vi "Scalar JSON text to Variant.vi"(6 "Type":T1, 8 "error in (no error)":errorcluster, 9 "Variant (Data Type)":variant, 10 "Offset (no whitespace)":i32, 11 "JSON":string) -> (0 "error out":errorcluster, 1 "Variant out":variant)   [LabVIEW 2024, in "JSONtext.lvlib"]
uses:
  JSONtext.lvlib
  Data Type.ctl
  Parsing State.ctl
  Refnum Type.ctl
  Advance past String.vi
  String Subset.vi
  Strip Quotes and Unescape.vi
  Get Number Text.vi
  NaN or null to Integer ERROR.vi
  Advance past Number.vi
  Unescape JSON string.vi
  Advance past Line Ending.vi
  Text to Timestamp.vi
  NI_Data Type.lvlib
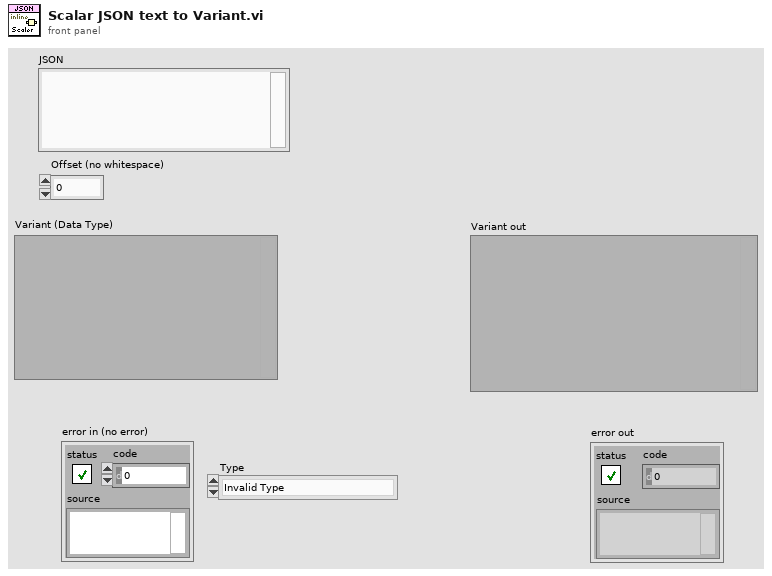
[diagram p1: front panel]
types:
  T1 = typedef "NI_Data Type.lvlib/Data Type.ctl" = enum8{"Invalid Type", "Void", "I8", "I16", "I32", "I64", "U8", "U16", "U32", "U64", "Single Float", "Double Float", "Extended Float", "Single Complex", "Double Complex", "Extended Complex", "Enum U8", "Enum U16", "Enum U32", "Enum U64", "Single Float With Unit", "Double Float With Unit", "Extended Float With Unit", "Single Complex with Unit", "Double Complex with Unit", "Extended Complex with Unit", "Boolean", "String", "Path", "Picture", "Tag", "Array", "Cluster", "Variant", "LV Variant", "Waveform", "Timestamp", "Digital Waveform", "Digital Data", "ExpressData", "Refnum", "External Data", "VI", "Poly VI", "LabVIEW Class Instance", "Fixed Point", "Set Collection", "Map Collection"}
  T2 = typedef "JSONtext.lvlib/Parsing State.ctl" = enum16{"Parser Error", "Object", "Array", "String", "Number/Other", "Leading Whitespace", "Object end", "Array end", "Value end"}
  T3 = typedef "NI_Data Type.lvlib/Refnum Type.ctl" = enum16{"NotARefnum", "UnknownRefnum", "Generic", "Datalog", "ByteStream", "Device", "Occurence", "TCPNetConnection", "Auto", "Menu", "Imaq", "Hardware", "DataSocket", "Visa", "IVI", "UDPNetConnection", "Notifier", "Queue", "Irda", "EventReg", "DotNet", "UserEvent", "Callback", "UNUSED_EMPTY_POSITION", "BlueToothNetConnection", "LVObjApp", "LVObjVI", "LVObjUnknown", "GenericClass", "UserDefinedRefnumTag", "DataValue", "RT FIFO", "TDMS File", "PythonSessionRefnum"}
  T4 = typedef "JSONtext.lvlib/JSON Value Type.ctl" = enum16{"Not a JSON Value", "JSON Object", "JSON Array", "String", "Number", "true", "false", "null"}
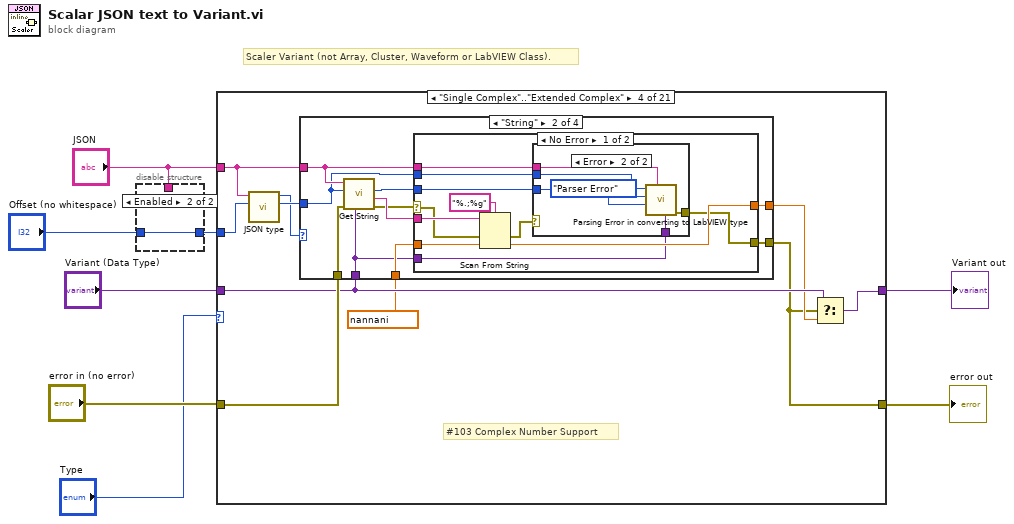
[diagram p0: block diagram]
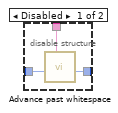
[diagram p2: hidden frame]
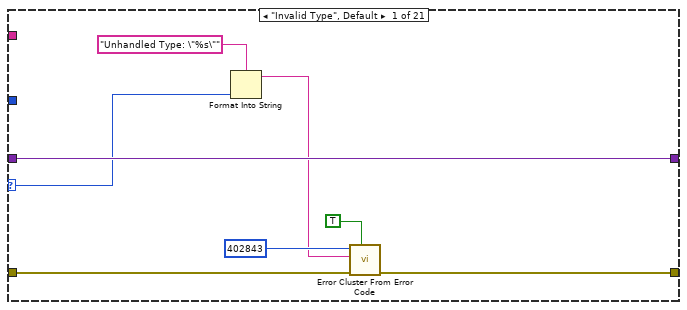
[diagram p3: hidden frame]
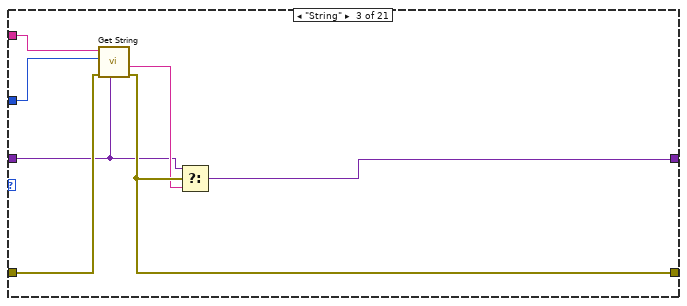
[diagram p5: hidden frame]
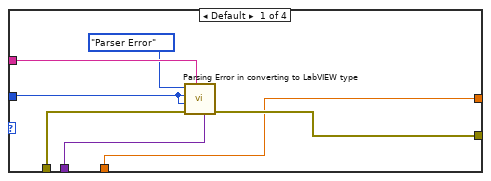
[diagram p6: hidden frame]
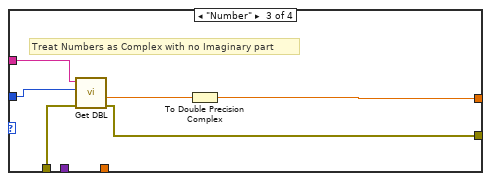
[diagram p9: hidden frame]
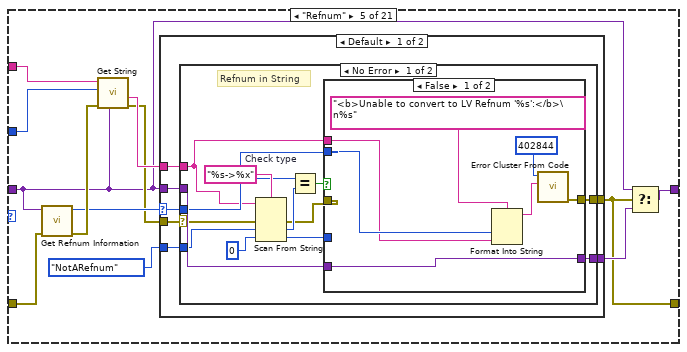
[diagram p11: hidden frame]
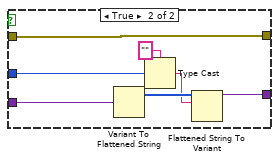
[diagram p12: hidden frame]
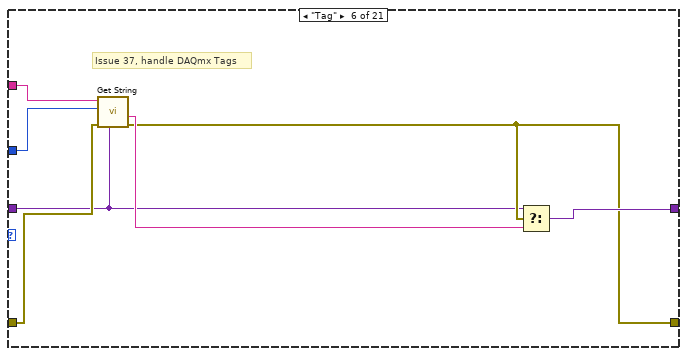
[diagram p15: hidden frame]
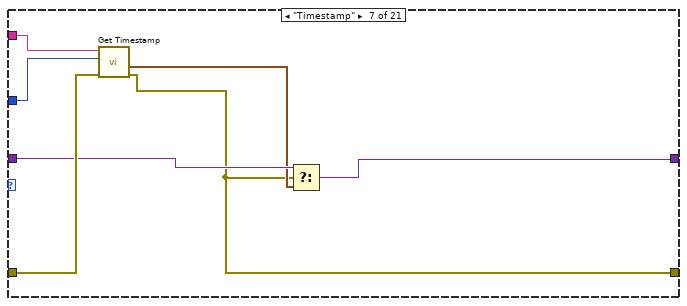
[diagram p16: hidden frame]
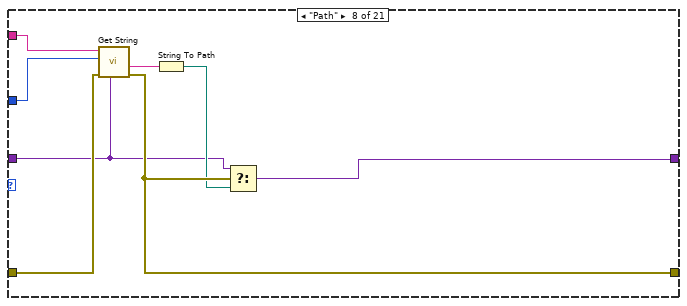
[diagram p17: hidden frame]
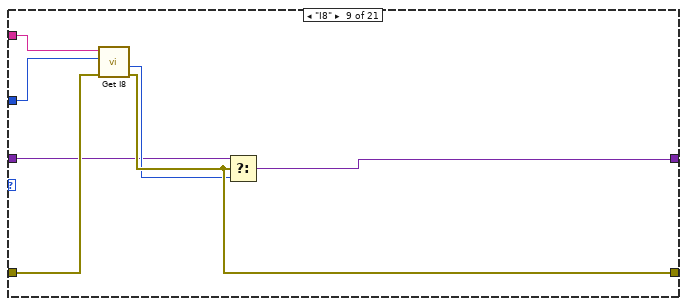
[diagram p18: hidden frame]
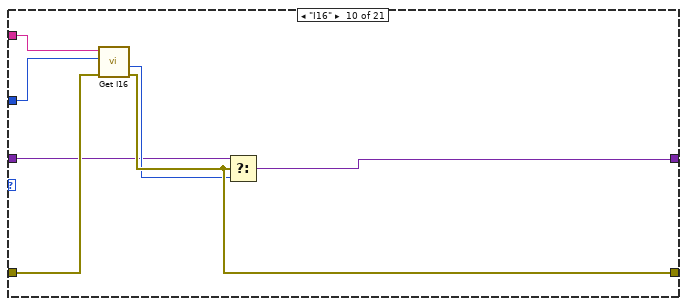
[diagram p19: hidden frame]
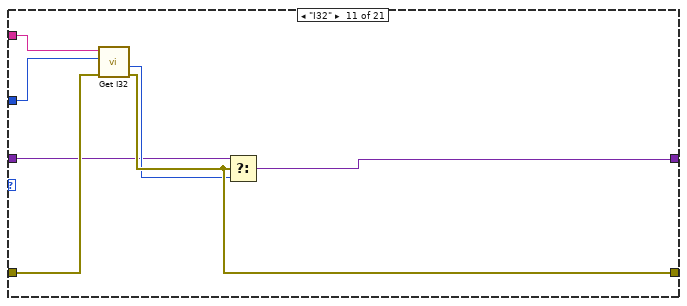
[diagram p20: hidden frame]
diagram:
  # "Scaler Variant (not Array, Cluster, Waveform or LabVIEW Class)."
  n1 = disable-structure shown="Enabled" {
    disable-tunnel: "Offset (no whitespace)" -> [w11 w12]
    disable-tunnel: [w10 w12] -> w4
    disable-tunnel: "JSON" -> [w9 _]
    frame Disabled {
      n2 = call "Advance past whitespace.vi"("JSON"=w9, "Offset"=w11) -> ("Offset of first non-whitespace"=w10:i32)  [unwired: 7 in, 2 out]
    }
    frame Enabled {
    }
  }
  n3 = case shown="\"Single Complex\"..\"Extended Complex\"" "Type" {
    selector: "Type" -> [w15 _ _ _ _ _ _ _ _ _ _ _ _ _ _ _ _ w219 _ _ _]
    tunnel: "Variant (Data Type)" -> [w19 w21 w23 w37 w85 w134 w144 w148 w156 w163 w170 w177 w184 w191 w198 w205 w216 w220 w249 w258 w271]
    tunnel: "JSON" -> [_ _ w28 w35 w95 w139 w146 w154 w158 w165 w172 w179 w186 w193 w200 w207 w213 w228 w246 w254 w268]
    tunnel: [w18 w22 w25 w31 w87 w135 w141 w151 w159 w166 w173 w180 w187 w194 w201 w208 w214 w224 w247 w252 w269] -> w7
    tunnel: "error in (no error)" -> [w20 w22 w27 w39 w93 w137 w145 w153 w161 w168 w175 w182 w189 w196 w203 w210 w217 w229 w250 w259 w272]
    tunnel: w4 -> [_ _ w29 w34 w96 w140 w147 w155 w162 w169 w176 w183 w190 w197 w204 w211 w218 w230 w251 w260 w273]
    tunnel: [w19 w21 w26 w38 w94 w138 w143 w152 w160 w167 w174 w181 w188 w195 w202 w209 w215 w225 w248 w257 w270] -> w6
    frame "Invalid Type", Default {
      n4 = Format Into String(format string="Unhandled Type: \"%s\"", w15) -> (resulting string=w13:string)  [unwired: 2 in, 1 out]
      n5 = call "Error Cluster From Error Code.vi"("show call chain? (False)"=TRUE, "error in (no error)"=w20, "error message (\"\")"=w13, "error code (0)"=402843) -> ("error out"=w18:errorcluster)  [unwired: 5 in]
    }
    frame "Void" {
      # "Empty Variant: #ToDo Variant Attributes?"
    }
    frame "String" {
      n6 = call "Get String.vi"("LV Type"=w23, "error in (no error)"=w27, "Offset"=w29, "JSON"=w28) -> ("error out"=w25:errorcluster, "String"=w24:string)  [unwired: 5 in, 1 out]
      n7 = Select(t=w23, s=w25, f=w24) -> (s? t:f=w26:variant)
    }
    frame "Single Complex".."Extended Complex" {
      # "#103 Complex Number Support"
      n8 = call "JSON type.vi"("Offset"=w34, "JSON"=w35) -> ("Item Offset"=w33:i32, "JSON Value Type"=w32:T4)  [unwired: 8 in]
      n9 = case shown="\"String\"" w32 {
        tunnel: w39 -> [w43 w56 w80 w84]
        tunnel: w37 -> [w44 w47 _ _]
        tunnel: [w40 w54 w78 w83] -> w36
        tunnel: w35 -> [w46 w52 w82 _]
        tunnel: w33 -> [w42 w50 w81 _]
        tunnel: [w41 w48 w77 w84] -> w31
        tunnel: cdb nan+nani ("default value 1") -> [w40 w53 _ w83]
        frame Default {
          n10 = call "Parsing Error in converting to LabVIEW type.vi"("LV Type"=w44, "JSON"=w46, "error in (no error)"=w43, "Offset past match"=w42, "Value start"=w42, "State"=Parsing_State."Parser Error") -> ("error out"=w41:errorcluster)  [unwired: 5 in]
        }
        frame "String" {
          n11 = call "Get String.vi"("LV Type"=w47, "error in (no error)"=w56, "Offset"=w50, "JSON"=w52) -> ("error out"=w49:errorcluster, "String"=w55:string, "Offset past match"=w51:i32)  [unwired: 5 in]
          n12 = case shown="No Error" w49 {
            selector: w49 -> [w58 w76]
            tunnel: w55 -> [w67 _]
            tunnel: [w66 w75] -> w54
            tunnel: w53 -> [w64 w75]
            tunnel: w52 -> [w63 _]
            tunnel: w51 -> [w62 _]
            tunnel: w50 -> [w61 _]
            tunnel: [w59 w76] -> w48
            tunnel: w47 -> [w57 _]
            frame No Error {
              n13 = Scan From String(format string="%.;%g", input string=w67, error in=w58, default 1=w64) -> (error out=w60:errorcluster, output 1=w66:cdb)  [unwired: 1 in, 2 out]
              n14 = case shown="Error" w60 {
                selector: w60 -> [w68 _]
                tunnel: w63 -> [_ w74]
                tunnel: w62 -> [_ w73]
                tunnel: w61 -> [_ w72]
                tunnel: [w68 w70] -> w59
                tunnel: w57 -> [_ w69]
                frame No Error {
                }
                frame Error {
                  n15 = call "Parsing Error in converting to LabVIEW type.vi"("LV Type"=w69, "JSON"=w74, "Offset past match"=w73, "Value start"=w72, "State"=Parsing_State."Parser Error") -> ("error out"=w70:errorcluster)  [unwired: 6 in]
                }
              }
            }
            frame Error {
            }
          }
        }
        frame "Number" {
          # "Treat Numbers as Complex with no Imaginary part"
          n16 = call "Get DBL.vi"("error in (no error)"=w80, "Offset"=w81, "JSON"=w82) -> ("error out"=w77:errorcluster, "Number"=w79:dbl)  [unwired: 6 in, 1 out]
          n17 = To Double Precision Complex(1:w79) -> (0:w78:cdb)
        }
        frame "null" {
          # "null == NaN"
        }
      }
      n18 = Select(t=w37, s=w31, f=w36) -> (s? t:f=w38:variant)
    }
    frame "Refnum" {
      n19 = call "Get Refnum Information.vi"("error in (no error)"=w93, "variant"=w85) -> ("error out"=w92:errorcluster, "reference type"=w91:T3)  [unwired: 6 in, 2 out]
      n20 = call "Get String.vi"("LV Type"=w85, "error in (no error)"=w92, "Offset"=w96, "JSON"=w95) -> ("error out"=w88:errorcluster, "String"=w89:string)  [unwired: 5 in, 1 out]
      n21 = case shown="Default" w91 {
        selector: w91 -> [w97 _]
        tunnel: [w102 w133] -> w90
        tunnel: w89 -> [w99 w133]
        tunnel: w85 -> [w103 _]
        tunnel: w88 -> [w101 w132]
        tunnel: [w100 w132] -> w87
        tunnel: Refnum_Type."NotARefnum" ("Reference Type") -> [w98 _]
        frame Default {
          n22 = case shown="No Error" w101 {
            selector: w101 -> [w111 w131]
            tunnel: w103 -> [w116 _]
            tunnel: [w115 _] -> w102
            tunnel: [w106 w131] -> w100
            tunnel: w99 -> [w104 _]
            tunnel: w98 -> [w110 _]
            tunnel: w97 -> [w105 _]
            frame No Error {
              # "Refnum in String"
              n23 = Scan From String(format string="%s->%x", input string=w104, error in=w111, default 1=w110, default 2=u32 0) -> (error out=w107:errorcluster, output 1=w109:T3, output 2=w112:u32)  [unwired: 1 in, 2 out]
              n24 = Equal? "Check type"(x=w105, y=w109) -> (x = y?=w108:bool)
              n25 = case shown="False" w108 {
                tunnel: w116 -> [w123 w128]
                tunnel: [w123 w127] -> w115
                tunnel: w112 -> [_ w125]
                tunnel: w107 -> [_ w124]
                tunnel: [w122 w124] -> w106
                tunnel: w105 -> [w118 _]
                tunnel: w104 -> [w117 _]
                frame False {
                  n26 = Format Into String(format string="<b>Unable to convert to LV Refnum '%s':</b>\n%s", w118, w117) -> (resulting string=w120:string)  [unwired: 2 in, 1 out]
                  n27 = call "Error Cluster From Code.vi"("error message (\"\")"=w120, "error code (402840+)"=402844) -> ("error out"=w122:errorcluster)  [unwired: 7 in]
                }
                frame True {
                  n28 = Variant To Flattened String(Variant=w128) -> (1:w130:i16[])  [unwired: 1 out]
                  n29 = Type Cast(type="", x=w125) -> (*(type *) &x=w129:string)
                  n30 = Flattened String To Variant(6:w129, 7:w130) -> (3:w127:variant)  [unwired: 1 in, 1 out]
                }
              }
            }
            frame Error {
            }
          }
        }
        frame "Visa", "IVI", "UserDefinedRefnumTag" {
        }
      }
      n31 = Select(t=w85, s=w87, f=w90) -> (s? t:f=w94:variant)
    }
    frame "Tag" {
      # "Issue 37, handle DAQmx Tags"
      n32 = call "Get String.vi"("LV Type"=w134, "error in (no error)"=w137, "Offset"=w140, "JSON"=w139) -> ("error out"=w135:errorcluster, "String"=w136:string)  [unwired: 5 in, 1 out]
      n33 = Select(t=w134, s=w135, f=w136) -> (s? t:f=w138:variant)
    }
    frame "Timestamp" {
      n34 = call "Get Timestamp.vi"("error in (no error)"=w145, "Offset"=w147, "JSON"=w146) -> ("error out"=w141:errorcluster, "Timestamp"=w142:timestamp)  [unwired: 6 in, 1 out]
      n35 = Select(t=w144, s=w141, f=w142) -> (s? t:f=w143:variant)
    }
    frame "Path" {
      n36 = call "Get String.vi"("LV Type"=w148, "error in (no error)"=w153, "Offset"=w155, "JSON"=w154) -> ("error out"=w151:errorcluster, "String"=w149:string)  [unwired: 5 in, 1 out]
      n37 = String To Path(string=w149) -> (path=w150:path)
      n38 = Select(t=w148, s=w151, f=w150) -> (s? t:f=w152:variant)
    }
    frame "I8" {
      n39 = call "Get I8.vi"("error in (no error)"=w161, "Offset"=w162, "JSON"=w158) -> ("error out"=w159:errorcluster, "Number"=w157:i8)  [unwired: 6 in, 1 out]
      n40 = Select(t=w156, s=w159, f=w157) -> (s? t:f=w160:variant)
    }
    frame "I16" {
      n41 = call "Get I16.vi"("error in (no error)"=w168, "Offset"=w169, "JSON"=w165) -> ("error out"=w166:errorcluster, "Number"=w164:i16)  [unwired: 6 in, 1 out]
      n42 = Select(t=w163, s=w166, f=w164) -> (s? t:f=w167:variant)
    }
    frame "I32" {
      n43 = call "Get I32.vi"("error in (no error)"=w175, "Offset"=w176, "JSON"=w172) -> ("error out"=w173:errorcluster, "Number"=w171:i32)  [unwired: 6 in, 1 out]
      n44 = Select(t=w170, s=w173, f=w171) -> (s? t:f=w174:variant)
    }
    frame "I64" {
      n45 = call "Get I64.vi"("error in (no error)"=w182, "Offset"=w183, "JSON"=w179) -> ("error out"=w180:errorcluster, "Number"=w178:i64)  [unwired: 6 in, 1 out]
      n46 = Select(t=w177, s=w180, f=w178) -> (s? t:f=w181:variant)
    }
    frame "U8" {
      n47 = call "Get U8.vi"("error in (no error)"=w189, "Offset"=w190, "JSON"=w186) -> ("error out"=w187:errorcluster, "Number"=w185:u8)  [unwired: 6 in, 1 out]
      n48 = Select(t=w184, s=w187, f=w185) -> (s? t:f=w188:variant)
    }
    frame "U16" {
      n49 = call "Get U16.vi"("error in (no error)"=w196, "Offset"=w197, "JSON"=w193) -> ("error out"=w194:errorcluster, "Number"=w192:u16)  [unwired: 6 in, 1 out]
      n50 = Select(t=w191, s=w194, f=w192) -> (s? t:f=w195:variant)
    }
    frame "U32" {
      n51 = call "Get U32.vi"("error in (no error)"=w203, "Offset"=w204, "JSON"=w200) -> ("error out"=w201:errorcluster, "Number"=w199:u32)  [unwired: 6 in, 1 out]
      n52 = Select(t=w198, s=w201, f=w199) -> (s? t:f=w202:variant)
    }
    frame "U64" {
      n53 = call "Get U64.vi"("error in (no error)"=w210, "Offset"=w211, "JSON"=w207) -> ("error out"=w208:errorcluster, "Number"=w206:u64)  [unwired: 6 in, 1 out]
      n54 = Select(t=w205, s=w208, f=w206) -> (s? t:f=w209:variant)
    }
    frame "Boolean" {
      n55 = call "Get Boolean.vi"("error in (no error)"=w217, "Offset"=w218, "JSON"=w213) -> ("error out"=w214:errorcluster, "Boolean"=w212:bool)  [unwired: 6 in, 1 out]
      n56 = Select(t=w216, s=w214, f=w212) -> (s? t:f=w215:variant)
    }
    frame "Enum U8".."Enum U64" {
      # "I32, but enums never bigger than that"
      n57 = call "Get String.vi"("LV Type"=w220, "error in (no error)"=w229, "Offset"=w230, "JSON"=w228) -> ("error out"=w222:errorcluster, "String"=w223:string)  [unwired: 5 in, 1 out]
      n58 = call "Get Numeric Information.vi"("error in (no error)"=w222, "variant"=w220) -> ("error out"=w221:errorcluster, "enum names"=w226:string[])  [unwired: 6 in, 2 out]
      n59 = Search 1D Array(1D array=w226, element=w223) -> (index of element=w227:i32)  [unwired: 1 in]
      n60 = case shown="0.." w227 {
        selector: w227 -> [w234 _]
        tunnel: [w233 w239] -> w225
        tunnel: w220 -> [w235 w239]
        tunnel: w221 -> [w232 w242]
        tunnel: [w231 w244] -> w224
        tunnel: w223 -> [_ w237]
        tunnel: w219 -> [w236 _]
        frame 0.. {
          n61 = call "Coerce I32 to Variant Intger.vi"("error in (no error)"=w232, "Type"=w236, "Default in"=w235, "I32"=w234) -> ("error out"=w231:errorcluster, "Variant (Data Type) out"=w233:variant)  [unwired: 6 in]
        }
        frame ..-1 {
          n62 = call "Get Type Information.vi"("variant"=w239) -> ("name"=w238:string)  [unwired: 6 in, 4 out]
          n63 = Format Into String(format string="Unknown Enum element \"%s\" for '%s'", w237, w238) -> (resulting string=w240:string)  [unwired: 2 in, 1 out]
          n64 = call "Error Cluster From Error Code.vi"("error in (no error)"=w242, "error message (\"\")"=w240, "error code (0)"=402844) -> ("error out"=w244:errorcluster)  [unwired: 6 in]
        }
      }
    }
    frame "Double Float", "Extended Float", "Double Float With Unit", "Extended Float With Unit" {
      # "Note: LabVIEW string functions can't really handle greater than DBL\nprecision, so we arn't really supporting EXT.  Consider alternate parsing in future."
      n65 = call "Get DBL.vi"("error in (no error)"=w250, "Offset"=w251, "JSON"=w246) -> ("error out"=w247:errorcluster, "Number"=w245:dbl)  [unwired: 6 in, 1 out]
      n66 = Select(t=w249, s=w247, f=w245) -> (s? t:f=w248:variant)
    }
    frame "Fixed Point" {
      # "NaN --> default"
      # "Issue 31 Fixed Point"
      n67 = call "Get DBL.vi"("error in (no error)"=w259, "Offset"=w260, "JSON"=w254) -> ("error out"=w255:errorcluster, "Number"=w256:dbl)  [unwired: 6 in, 1 out]
      n68 = Not A Number/Path/Refnum?(number/path/refnum=w256) -> (NaN/Path/Refnum?=w253:bool)
      n69 = case shown="True" w253 {
        tunnel: w255 -> [w261 w266]
        tunnel: [w261 w265] -> w252
        tunnel: w254 -> [_ w262]
        frame False {
        }
        frame True {
          n70 = call "Format Error.vi"("error code (402842)"=402844, "error in (no error)"=w266, "message part 2"=w262, "error message"="Cannot Get as Fixed Point: " ("format string")) -> ("error out"=w265:errorcluster)  [unwired: 7 in]
        }
      }
      n71 = Select(t=w258, s=w252, f=w256) -> (s? t:f=w257:variant)
    }
    frame "Single Float", "Single Float With Unit" {
      n72 = call "Get SGL.vi"("error in (no error)"=w272, "Offset"=w273, "JSON"=w268) -> ("error out"=w269:errorcluster, "Number"=w267:sgl)  [unwired: 6 in, 1 out]
      n73 = Select(t=w271, s=w269, f=w267) -> (s? t:f=w270:variant)
    }
  }
  "Variant out" <- w6
  "error out" <- w7
